vi "Create New VI or CTL From Template.vi"(8 "error in":errorcluster, 10 "Selected Template VI or CTL name (including file extension)":string, 11 "Destination Folder":path) -> (0 "error out":errorcluster, 3 "Reference of newly created VI":refnum<vi>)   [LabVIEW 2021]
doc: "Creates a new VI or CTL as a \"Save as...\" copy of a template."
panel:
  # "Development\ncontrols/indicators useful for development and testing, but which are not outputs of the VI"
  # "Input\nInputs to the VI"
  # "Output\nOutputs of the VI"
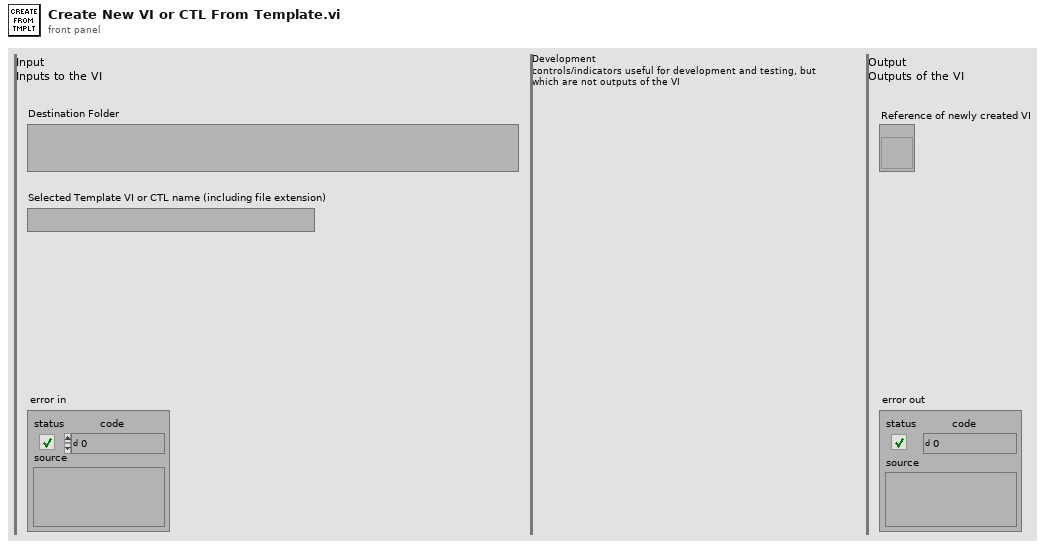
[diagram p1: front panel]
types:
  T1 = enum32{"invalid VI type", "Standard VI", "Control VI", "Global VI", "Polymorphic VI", "Configuration VI", "SubSystem", "Facade VI", "Method VI", "Statechart Diagram VI"}
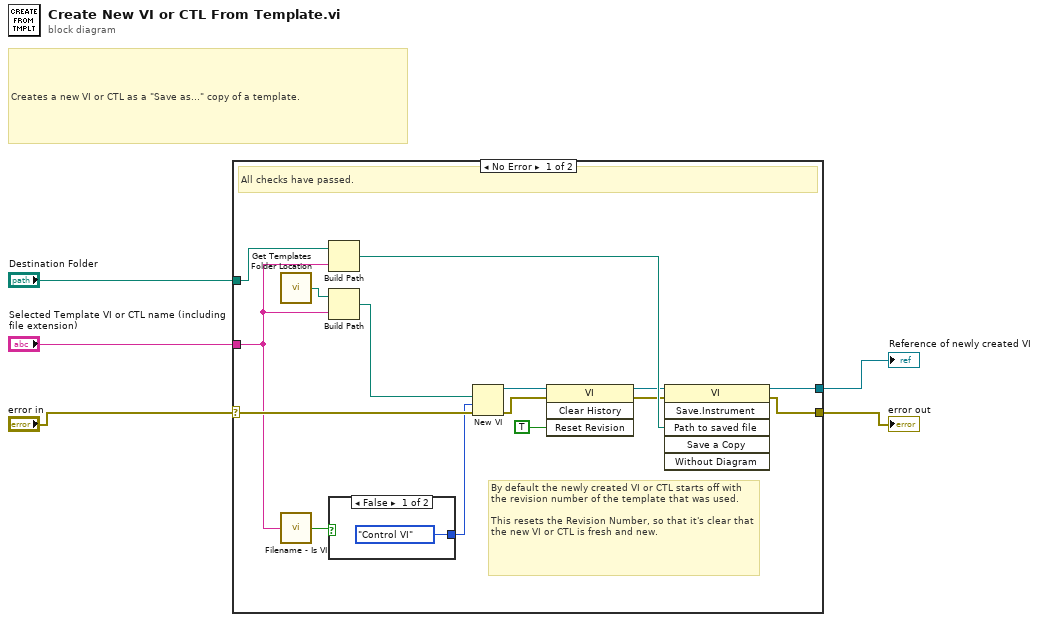
[diagram p0: block diagram]
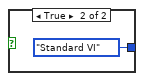
[diagram p2: hidden frame]
diagram:
  # "Creates a new VI or CTL as a \"Save as...\" copy of a template."
  n1 = case shown="No Error" "error in" {
    selector: "error in" -> [w19 w23]
    tunnel: [w16 w23] -> w4
    tunnel: "Selected Template VI or CTL name (including file extension)" -> [w13 _]
    tunnel: "Destination Folder" -> [w20 _]
    tunnel: [w6 _] -> w1
    frame No Error {
      # "By default the newly created VI or CTL starts off with the revision number of the template that was used.\n\nThis resets the Revision Number, so that it's clear that the new VI or CTL is fresh and new."
      # "All checks have passed."
      n2 = call "Get Templates Folder Location.vi"() -> ("Templates Folder Location"=w18:path)
      n3 = call "Filename - Is VI.vi"("Filename (including file extension)"=w13) -> ("Is VI?"=w12:bool)
      n4 = Build Path(base path=w20, name or relative path=w13) -> (appended path=w15:path)
      n5 = Build Path(base path=w18, name or relative path=w13) -> (appended path=w17:path)
      n6 = case shown="False" w12 {
        tunnel: [T1."Control VI" ("vi type (standard vi)") T1."Standard VI" ("vi type (standard vi)")] -> w14
        frame False {
        }
        frame True {
        }
      }
      n7 = New VI(8:w19, 9:w14, 10:w17) -> (0:w10:errorcluster, 3:w11:refnum<vi>)  [unwired: 4 in]
      n8 = invoke class="VI" method="Clear History"(reference=w11, error in=w10, "Reset Revision"=TRUE) -> (reference out=w8:refnum<vi>, error out=w9:errorcluster)  [unwired: 1 in, 2 out]
      n9 = invoke class="VI" method="Save.Instrument"(reference=w8, error in=w9, "Path to saved file"=w15) -> (reference out=w6:refnum<vi>, error out=w16:errorcluster)  [unwired: 3 in, 4 out]
    }
    frame Error {
      # "Do nothing. The error message will be handled later, downstream"
      # "One or more checks failed."
    }
  }
  "error out" <- w4
  "Reference of newly created VI" <- w1
